vi "ELOG_TimestampFormat_Set.vi"(8 "error in (no error)":errorcluster, 10 "Timestamp Format":T1, 11 "OXY_SCPI Reseource In":refnum<visa-resource-name>) -> (0 "error out":errorcluster, 1 "communication_data":T2, 3 "OXY_SCPI Reseource Out":refnum<visa-resource-name>)   [LabVIEW 2018, in "OXYGEN.lvlib"]
doc: "Sets the requested timestamp format"
uses:
  OXYGEN.lvlib
  TypeDefs/Cluster_RawCommData.ctl
  TypeDefs/Enum_ELOGtimeFormats.ctl
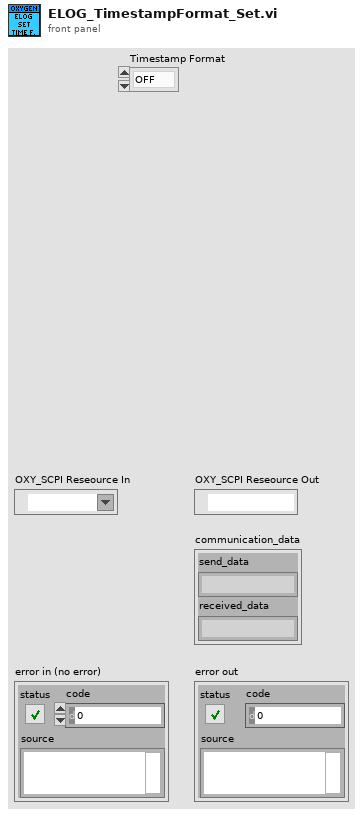
[diagram p1: front panel]
types:
  T1 = typedef "OXYGEN.lvlib/Enum_ELOGtimeFormats.ctl" = enum16{"OFF", "REL", "ELOG", "ABS"}
  T2 = typedef "OXYGEN.lvlib/Cluster_RawCommData.ctl" = cluster{"send_data":string, "received_data":string}
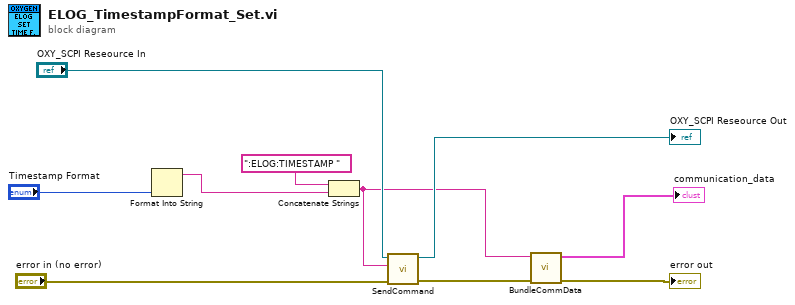
[diagram p0: block diagram]
diagram:
  n1 = Format Into String("Timestamp Format") -> (resulting string=w2:string)  [unwired: 3 in, 1 out]
  n2 = Concatenate Strings(":ELOG:TIMESTAMP " ("string"), w2) -> (w7:string)
  n3 = call "SendCommand.vi"("error in (no error)"="error in (no error)", "String to Send"=w7, "OXY_SCPI Reseource In"="OXY_SCPI Reseource In") -> ("error out"=w4:errorcluster, "OXY_SCPI Reseource Out"=→"OXY_SCPI Reseource Out":refnum<visa-resource-name>)  [unwired: 7 in]
  n4 = call "BundleCommData.vi"("error in (no error)"=w4, "send_data"=w7) -> ("error out"=→"error out":errorcluster, "communication_data"=→"communication_data":T2)  [unwired: 8 in]
